vi "ReceiveCrossingEvent.vi"(0 "channel":u16=1 min=1 max=8, 5 "clock offset":i64, 9 "socket in":refnum<class "zmq_socket.lvclass">, 11 "error in":errorcluster) -> (1 "threshold":sgl, 3 "rising?":bool, 4 "new crossing":bool, 6 "crossing time":i64, 8 "learning rate":dbl, 10 "socket out":refnum<class "zmq_socket.lvclass">, 12 "event time":i64, 14 "crossing level":sgl, 15 "error out":errorcluster)   [LabVIEW 2017]
uses:
  <vilib>/addons/zeromq/zmq_socket.lvclass
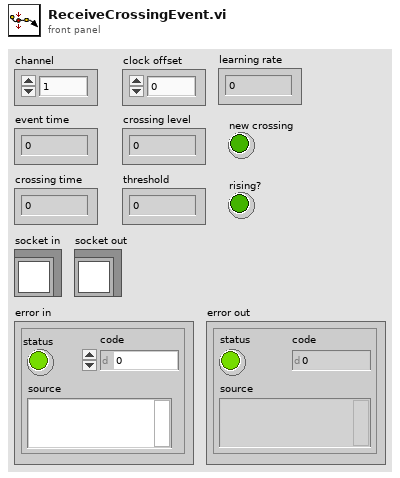
[diagram p1: front panel]
types:
  T1 = enum16{"big-endian, network order", "native, host order", "little-endian"}
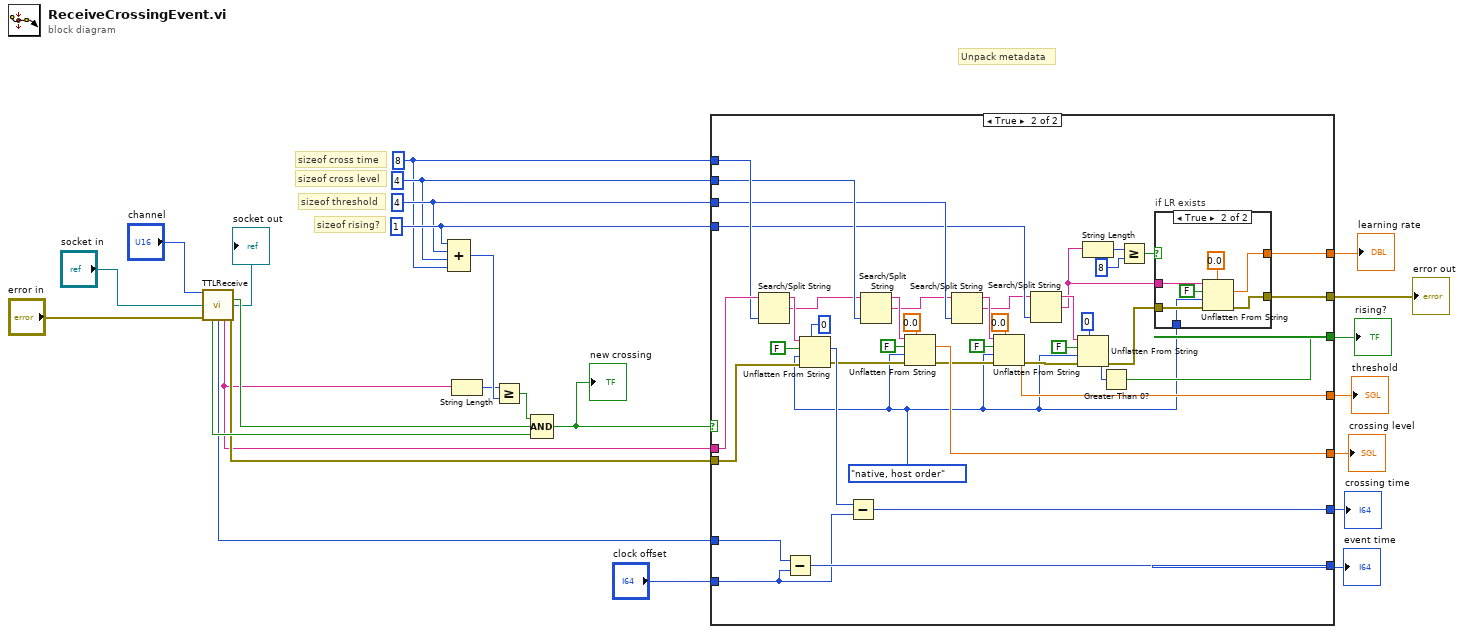
[diagram p0: block diagram]
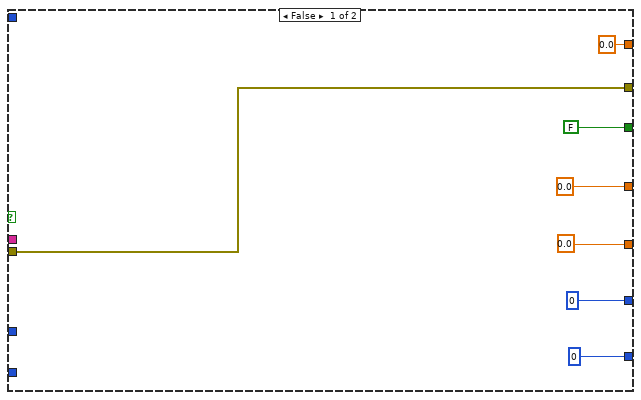
[diagram p2: hidden frame]
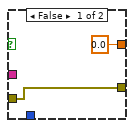
[diagram p3: hidden frame]
diagram:
  w8 = 1 ("offset (0)")
  w7 = 4 ("offset (0)")
  w6 = 4 ("offset (0)")
  w5 = 8 ("offset (0)")
  # "sizeof rising?"
  # "sizeof threshold"
  # "sizeof cross level"
  # "sizeof cross time"
  # "Unpack metadata"
  n1 = call "TTLReceive.vi"("channel"="channel", "socket in"="socket in", "error in"="error in") -> ("new TTL"=w22:bool, "socket out"=→"socket out":refnum<class "zmq_socket.lvclass">, "event on"=w21:bool, "timestamp"=w17:i64, "metadata"=w4:string, "error out"=w15:errorcluster)  [unwired: 7 in]
  n2 = Compound Arithmetic op=unknown(w8, w7, w6, w5) -> (w2:i32)
  n3 = String Length(string=w4) -> (length=w1:i32)
  n4 = Greater Or Equal?(x=w1, y=w2) -> (x >= y?=w3:bool)
  n5 = Compound Arithmetic op=AND(w3, w22, w21) -> (w19:bool)
  "new crossing" <- w19
  n6 = case shown="True" w19 {
    tunnel: "clock offset" -> [_ w69]
    tunnel: w17 -> [_ w73]
    tunnel: w4 -> [_ w71]
    tunnel: [i64 0 w72] -> w16
    tunnel: w15 -> [w28 w70]
    tunnel: [i64 0 w68] -> w14
    tunnel: [sgl 0.0 w67] -> w13
    tunnel: [sgl 0.0 w66] -> w12
    tunnel: [w28 w64] -> w11
    tunnel: [FALSE w65] -> w10
    tunnel: [0.0 w63] -> w9
    tunnel: w5 -> [_ w62]
    tunnel: w6 -> [_ w61]
    tunnel: w7 -> [_ w60]
    tunnel: w8 -> [_ w59]
    frame False {
    }
    frame True {
      w34 = T1."native, host order" ("byte order (0:big-endian, network order)")
      n7 = Search/Split String(string=w71, offset (0)=w62) -> (substring before match=w58:string, match + rest of string=w54:string)  [unwired: 1 in, 1 out]
      n8 = Subtract(x=w73, y=w69) -> (x-y=w72:i64)
      n9 = Unflatten From String(type=i64 0, binary string=w58, data includes array or string size? (T)=FALSE, byte order (0:big-endian, network order)=w34, error in (no error)=w70) -> (value=w55:i64, error out=w52:errorcluster)  [unwired: 1 out]
      n10 = Subtract(x=w55, y=w69) -> (x-y=w68:i64)
      n11 = Search/Split String(string=w54, offset (0)=w61) -> (substring before match=w53:string, match + rest of string=w49:string)  [unwired: 1 in, 1 out]
      n12 = Unflatten From String(type=sgl 0.0, binary string=w53, data includes array or string size? (T)=FALSE, byte order (0:big-endian, network order)=w34, error in (no error)=w52) -> (value=w67:sgl, error out=w47:errorcluster)  [unwired: 1 out]
      n13 = Search/Split String(string=w49, offset (0)=w60) -> (substring before match=w48:string, match + rest of string=w40:string)  [unwired: 1 in, 1 out]
      n14 = Unflatten From String(type=sgl 0.0, binary string=w48, data includes array or string size? (T)=FALSE, byte order (0:big-endian, network order)=w34, error in (no error)=w47) -> (value=w66:sgl, error out=w44:errorcluster)  [unwired: 1 out]
      n15 = Search/Split String(string=w40, offset (0)=w59) -> (substring before match=w39:string, match + rest of string=w33:string)  [unwired: 1 in, 1 out]
      n16 = Unflatten From String(type=u8 0, binary string=w39, data includes array or string size? (T)=FALSE, byte order (0:big-endian, network order)=w34, error in (no error)=w44) -> (value=w42:u8, error out=w35:errorcluster)  [unwired: 1 out]
      n17 = String Length(string=w33) -> (length=w38:i32)
      n18 = Greater Than 0?(x=w42) -> (x > 0?=w65:bool)
      n19 = Greater Or Equal?(x=w38, y=8) -> (x >= y?=w36:bool)
      n20 = case "if LR exists" shown="True" w36 {
        tunnel: w33 -> [_ w82]
        tunnel: w35 -> [w74 w80]
        tunnel: w34 -> [_ w79]
        tunnel: [w74 w77] -> w64
        tunnel: [0.0 w76] -> w63
        frame False {
        }
        frame True {
          n21 = Unflatten From String(type=0.0, binary string=w82, data includes array or string size? (T)=FALSE, byte order (0:big-endian, network order)=w79, error in (no error)=w80) -> (value=w76:dbl, error out=w77:errorcluster)  [unwired: 1 out]
        }
      }
    }
  }
  "event time" <- w16
  "crossing time" <- w14
  "crossing level" <- w13
  "threshold" <- w12
  "error out" <- w11
  "rising?" <- w10
  "learning rate" <- w9
